vi "SingleAcquisition.vi"(8 "error in (no error)":errorcluster, 10 "Image In":T1, 11 "Inovance_Camera in":refnum<class "Inovance_Camera.lvclass">) -> (0 "error out":errorcluster, 3 "Inovance_Camera out":refnum<class "Inovance_Camera.lvclass">)   [LabVIEW 2023, in "Inovance_Camera.lvlib" / "Inovance_Camera.lvclass"]
uses:
  Inovance_Camera.lvclass
  C:/Program Files/National Instruments/LabVIEW 2023/vi.lib/ActorFramework/Actor/Actor.lvclass
  <vilib>/vision/Image Controls.llb/IMAQ Image.ctl
  <vilib>/ActorFramework/Actor/Actor.lvclass/Actor.ctl
  Inovance_Camera.lvclass/Inovance_Camera.ctl
  Interfaces/AbstractInstrumentClasses/Cameras_LV/CameraComm Messages/Frame Ready Msg/Frame Ready Msg.lvclass/Frame Ready Msg.ctl
  <vilib>/ActorFramework/Message Enqueuer/Message Enqueuer.lvclass/Message Enqueuer.ctl
  <vilib>/ActorFramework/Message Enqueuer/Enqueue.vi
  Interfaces/AbstractInstrumentClasses/Cameras_LV/CameraComm Messages/Frame Ready Msg/Frame Ready Msg.lvclass
  C:/Program Files/National Instruments/LabVIEW 2023/vi.lib/ActorFramework/Message/Message.lvclass
  <vilib>/ActorFramework/Message Priority Queue/Priority Enqueue.vi
  <vilib>/vision/driver/NI_Vision_Acquisition_Software.lvlib
  <vilib>/ActorFramework/Actor/Actor.lvclass
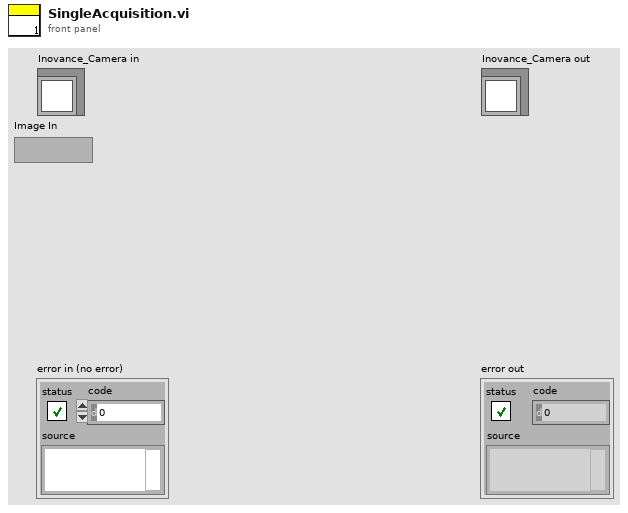
[diagram p1: front panel]
types:
  T1 = typedef "IMAQ Image.ctl" = refnum<image>
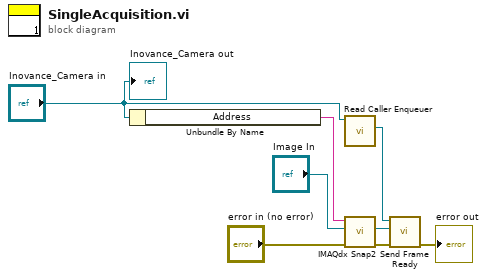
[diagram p0: block diagram]
diagram:
  n1 = Unbundle By Name("Inovance_Camera in") -> ("Address"=w8:string)
  n2 = call <vilib>:"Read Caller Enqueuer.vi"("Actor"="Inovance_Camera in") -> ("Caller Enqueuer"=w1:refnum<class "Message Enqueuer.lvclass">)  [unwired: 10 in]
  n3 = call <vilib>:"IMAQdx Snap2.vi"("error in"="error in (no error)", "Image In"="Image In", "Session In"=w8) -> ("error out"=w4:errorcluster, "Image Out"=w5:T1)  [unwired: 6 in, 1 out]
  n4 = call "Send Frame Ready.vi"("error in (no error)"=w4, "Image In"=w5, "Message Enqueuer"=w1) -> ("error out"=→"error out":errorcluster)  [unwired: 7 in, 1 out]
  "Inovance_Camera out" <- "Inovance_Camera in"
